vi "initialize.vi"(8 "Data Savefile Path":path=path "/home/lvuser/logs.bin", 9 "Refs Readfrom Path":path=path "/home/lvuser/logs.bin", 10 "RST Readfrom path":path=path "/home/lvuser/logs.bin", 11 "mode":T1=enum."pry_CL") -> (3 "Qube":refnum<class "System.lvclass">)   [LabVIEW 2021, in "System.lvclass"]
uses:
  System.lvclass
  mode.ctl
  System.lvclass/System.ctl
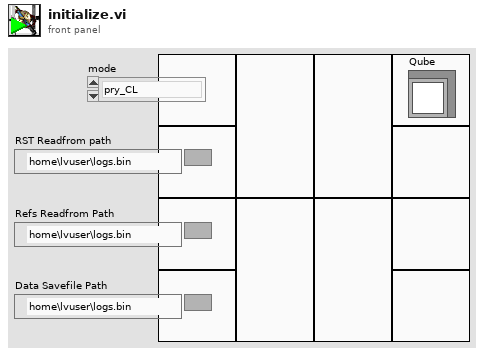
[diagram p1: front panel]
types:
  T1 = typedef "System.lvclass/mode.ctl" = enum16{"pry_OL", "pry_CL", "FBLR_CL"}
  T2 = enum16{"big-endian, network order", "native, host order", "little-endian"}
  T3 = enum16{"open", "replace", "create", "open or create", "replace or create", "replace or create with confirmation"}
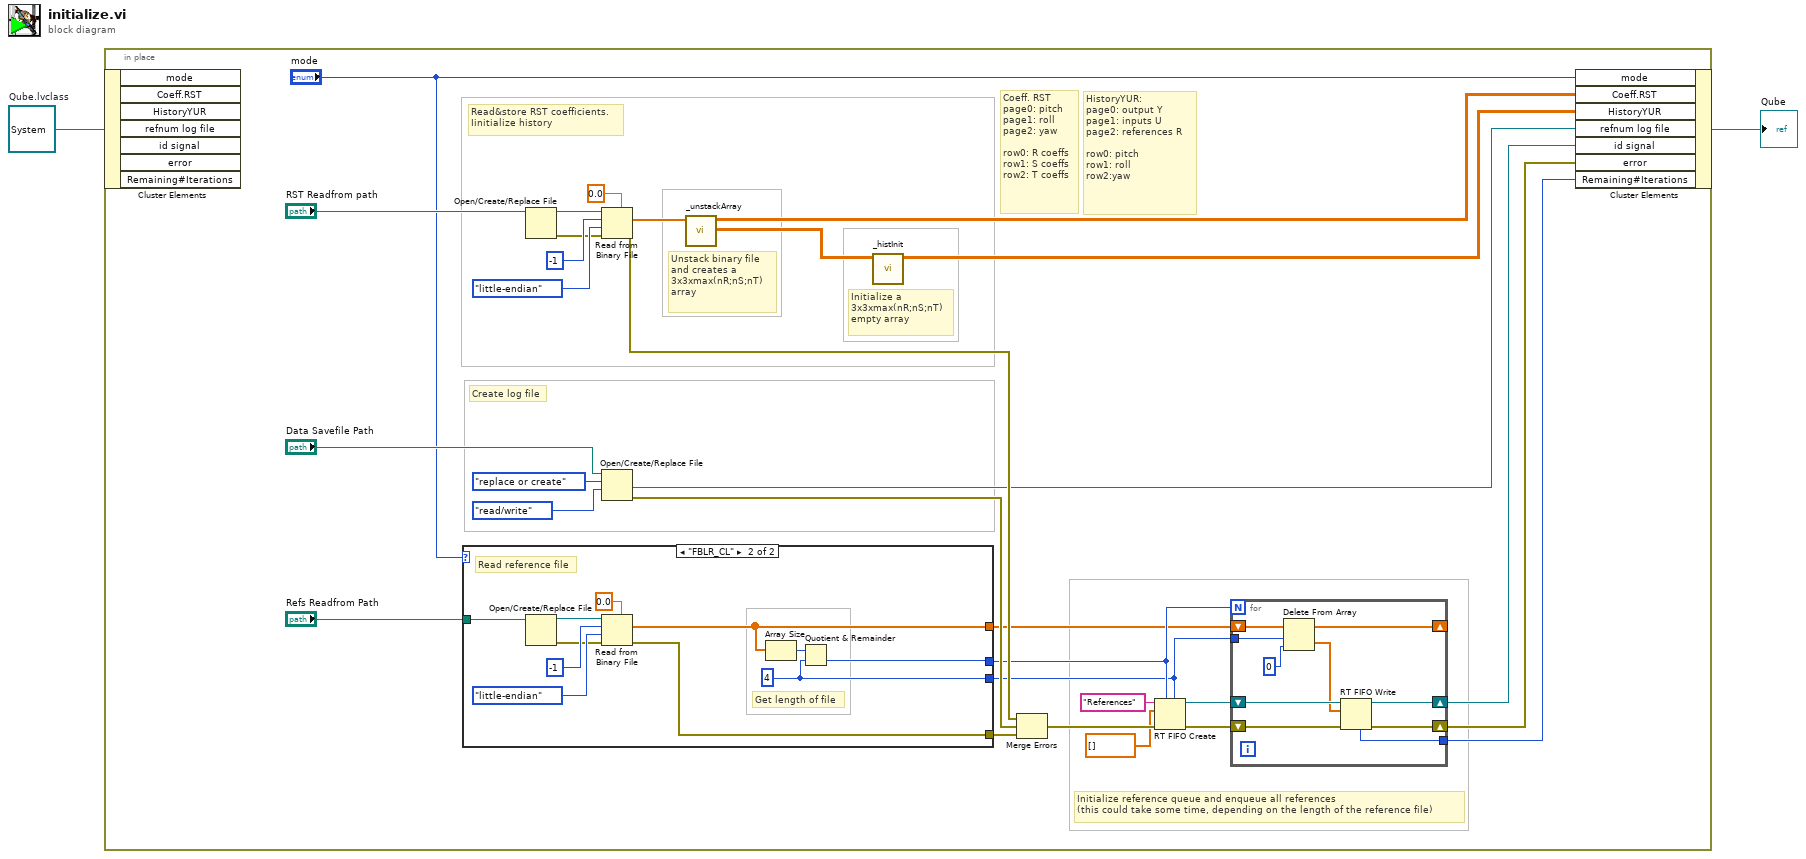
[diagram p0: block diagram]
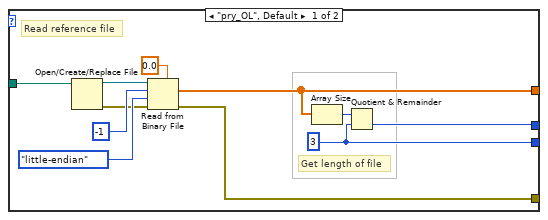
[diagram p2: hidden frame]
diagram:
  w1 = refnum<class "System.lvclass"> refnum  # Qube.lvclass
  n1 = in-place {
    # "Initialize reference queue and enqueue all references \n(this could take some time, depending on the length of the reference file)"
    # "Initialize a\n3x3xmax(nR;nS;nT)\nempty array"
    # "Coeff. RST\npage0: pitch\npage1: roll\npage2: yaw\n\nrow0: R coeffs\nrow1: S coeffs\nrow2: T coeffs"
    # "HistoryYUR:\npage0: output Y\npage1: inputs U\npage2: references R\n\nrow0: pitch\nrow1: roll\nrow2:yaw"
    # "Unstack binary file\nand creates a \n3x3xmax(nR;nS;nT) \narray"
    # "Read&store RST coefficients.\nIinitialize history"
    # "Create log file"
    n2 = in-place-cluster #1(w1) -> ()  [unwired: 7 out]
    n3 = case shown="\"FBLR_CL\"" "mode" {
      tunnel: [w47 w58] -> w29
      tunnel: "Refs Readfrom Path" -> [w49 w60]
      tunnel: [w43 w54] -> w11
      tunnel: [w45 w56] -> w3
      tunnel: [w44 w55] -> w12
      frame "pry_OL", Default {
        w43 = 3
        # "Get length of file"
        # "Read reference file"
        n4 = Open/Create/Replace File(file path (use dialog)=w49) -> (refnum out=w53:refnum<file>, error out=w48:errorcluster)  [unwired: 5 in, 1 out]
        n5 = Read from Binary File(5:0.0, 8:w48, 9:T2."little-endian" ("byte order (0:big-endian, network order)"), 10:-1 ("count (1)"), 11:w53) -> (0:w47:errorcluster, 2:w45:dbl[])  [unwired: 1 in, 2 out]
        n6 = Array Size(array=w45) -> (size(s)=w46:i32)
        n7 = Quotient & Remainder(x=w46, y=w43) -> (floor(x/y)=w44:i32)  [unwired: 1 out]
      }
      frame "FBLR_CL" {
        w54 = 4
        # "Get length of file"
        # "Read reference file"
        n8 = Open/Create/Replace File(file path (use dialog)=w60) -> (refnum out=w64:refnum<file>, error out=w59:errorcluster)  [unwired: 5 in, 1 out]
        n9 = Read from Binary File(5:0.0, 8:w59, 9:T2."little-endian" ("byte order (0:big-endian, network order)"), 10:-1 ("count (1)"), 11:w64) -> (0:w58:errorcluster, 2:w56:dbl[])  [unwired: 1 in, 2 out]
        n10 = Array Size(array=w56) -> (size(s)=w57:i32)
        n11 = Quotient & Remainder(x=w57, y=w54) -> (floor(x/y)=w55:i32)  [unwired: 1 out]
      }
    }
    n12 = Open/Create/Replace File(file path (use dialog)="RST Readfrom path") -> (refnum out=w26:refnum<file>, error out=w21:errorcluster)  [unwired: 5 in, 1 out]
    n13 = Read from Binary File(5:0.0, 8:w21, 9:T2."little-endian" ("byte order (0:big-endian, network order)"), 10:-1 ("count (1)"), 11:w26) -> (0:w20:errorcluster, 2:w19:dbl[])  [unwired: 1 in, 2 out]
    n14 = Open/Create/Replace File(file path (use dialog)="Data Savefile Path", operation (0:open)=T3."replace or create", access (0:read/write)=enum16{"read/write", "read-only", "write-only"}."read/write") -> (refnum out=w7:refnum<file>, error out=w28:errorcluster)  [unwired: 3 in, 1 out]
    n15 = call "_unstackArray.vi"("Stacked Array"=w19) -> ("Inner dimensions"=w18:dbl[][], "Unstacked Array"=w9:dbl[][][])  [unwired: 9 in]
    n16 = call "_histInit.vi"("RST Dimensions"=w18) -> ("YUR: history"=w8:dbl[][][])  [unwired: 10 in]
    n17 = Merge Errors(w20, w28, w29) -> (w17:errorcluster)
    n18 = RT FIFO Create(0:"References" ("name (unnamed)"), 1:dbl[] [], 3:w17, 4:w12, 6:w11) -> (8:w15:refnum<k33>, 11:w14:errorcluster)  [unwired: 3 in, 1 out]
    n19 = for {
      N: w12 -> [_]
      shift-right: [w39] -> w6
      shift-left: w15 -> [w42]
      shift-right: [w40] -> w5
      shift-left: w14 -> [w41]
      tunnel: w11 -> [w33]
      shift-right: [w36] -> _
      shift-left: w3 -> [w35]
      tunnel: [w34] -> w4
      n20 = Delete From Array(array=w35, length=w33, index=0) -> (deleted portion=w37:dbl[], array with subset deleted=w36:dbl[])
      n21 = RT FIFO Write(0:w42, 1:w37, 3:w41) -> (7:w34:u32, 8:w39:refnum<k33>, 11:w40:errorcluster)  [unwired: 2 in, 1 out]
    }
    n22 = in-place-cluster #1("mode"="mode", "Coeff.RST"=w9, "HistoryYUR"=w8, "refnum log file"=w7, "id signal"=w6, "error"=w5, "Remaining#Iterations"=w4) -> (→"Qube":refnum<class "System.lvclass">)
  }
